vi "释放引用.vi"(8 "error in (no error)":errorcluster caption="错误输入（无错误）", 11 "串口 输入":refnum<class "串口.lvclass"> caption="DNL_LabVIEW Object in") -> (0 "error out":errorcluster caption="错误输出", 3 "串口 输出":refnum<class "串口.lvclass"> caption="DNL_LabVIEW Object out")   [LabVIEW 2012, in "串口.lvclass"]
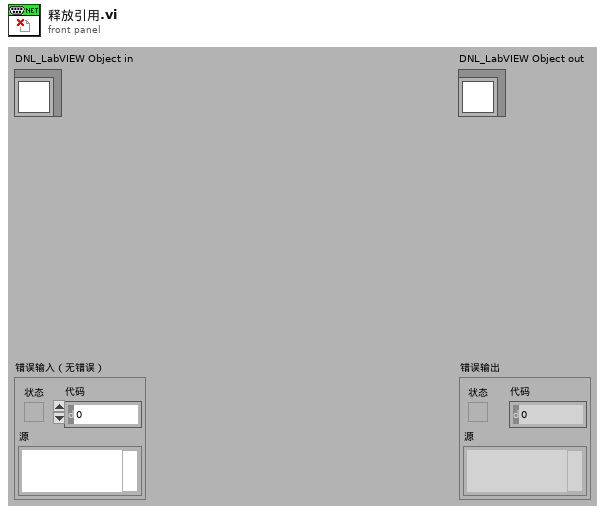
[diagram p1: front panel]
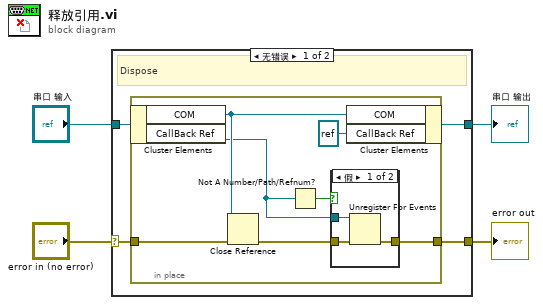
[diagram p0: block diagram]
diagram:
  n1 = case shown="无错误" "error in (no error)" {
    selector: "error in (no error)" -> [w6 w21]
    tunnel: [w5 w21] -> w3
    tunnel: [w7 w20] -> w1
    tunnel: "串口 输入" -> [w8 w20]
    frame No Error {
      # "Dispose"
      n2 = in-place {
        in-place-border: w6 -> [w14]
        in-place-border: [w10] -> w5
        n3 = in-place-cluster #1(w8) -> ("COM"=w15:refnum<k24>, "CallBack Ref"=w9:refnum<k27>)
        n4 = Close Reference(reference=w15, error in (no error)=w14) -> (error out=w11:errorcluster)
        n5 = Not A Number/Path/Refnum?(number/path/refnum=w9) -> (NaN/Path/Refnum?=w12:bool)
        n6 = case shown="假" w12 {
          tunnel: w11 -> [w18 w19]
          tunnel: [w17 w19] -> w10
          tunnel: w9 -> [w16 _]
          frame False {
            n7 = Unregister For Events(event registration refnum=w16, error in=w18) -> (error out=w17:errorcluster)
          }
          frame True {
          }
        }
        n8 = in-place-cluster #1("COM"=w15, "CallBack Ref"=refnum<k27> refnum) -> (w7:refnum<class "串口.lvclass">)
      }
    }
    frame Error {
    }
  }
  "error out" <- w3
  "串口 输出" <- w1
